vi "获取复合步骤名称XPath表达式.vi"(11 "查询参数":string) -> (3 "Union":string)   [LabVIEW 2022 SP3, in "斯坦道通用流路CODmn.lvlib"]
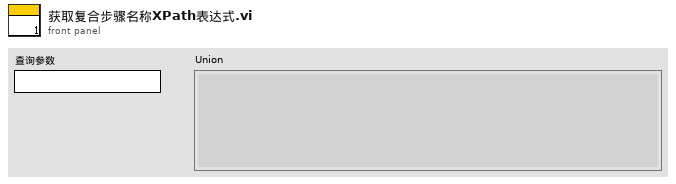
[diagram p1: front panel]
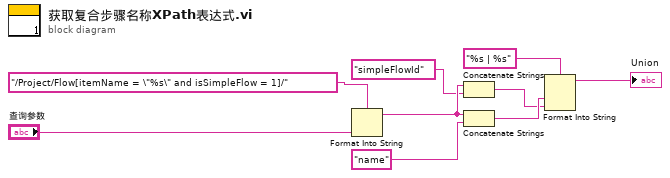
[diagram p0: block diagram]
diagram:
  n1 = Format Into String(format string="/Project/Flow[itemName = \"%s\" and isSimpleFlow = 1]/" ("格式字符串"), "查询参数") -> (resulting string=w6:string)  [unwired: 2 in, 1 out]
  n2 = Concatenate Strings(w6, "simpleFlowId" ("字符串")) -> (w2:string)
  n3 = Concatenate Strings(w6, "name" ("字符串")) -> (w3:string)
  n4 = Format Into String(format string="%s | %s" ("格式字符串"), w3, w2) -> (resulting string=→"Union":string)  [unwired: 2 in, 1 out]
